vi "GetFlattenedString.vi"(8 "error in":errorcluster, 11 "String in":refnum<class "String.lvclass">) -> (0 "error out":errorcluster, 2 "FlattenedString":string, 3 "String out":refnum<class "String.lvclass">)   [LabVIEW 2021, in "ProligentXMLGenerator.lvlib" / "String.lvclass"]
uses:
  String.lvclass
  String.lvclass/String.ctl
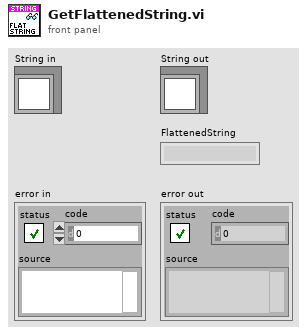
[diagram p1: front panel]
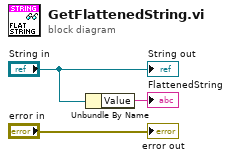
[diagram p0: block diagram]
diagram:
  n1 = Unbundle By Name("String in") -> ("Value"=→"FlattenedString":string)
  "error out" <- "error in"
  "String out" <- "String in"
